vi "Open file.vi"(0 "reference in":refnum<class "TDMS_DataHandler.lvclass">, 5 "error in (no error)":errorcluster) -> (14 "reference out":refnum<class "TDMS_DataHandler.lvclass">, 15 "tdms file out":refnum<k34>, 19 "error out":errorcluster)   [LabVIEW 2019, in "TDMS_DataHandler.lvclass"]
uses:
  TDMS_DataHandler.lvclass
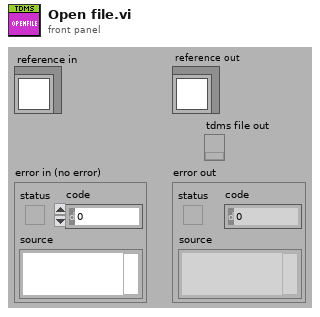
[diagram p1: front panel]
types:
  T1 = enum16{"open", "open or create", "create or replace", "create", "open (read-only)"}
  T2 = typedef "TDMS_DataHandler.lvclass/ObjectAttributesRef.ctl" = refnum<data-value>
  T3 = typedef "TDMS_DataHandler.lvclass/ObjectAttributes.ctl" = cluster{"Directory":path, "FilePath":path, "FileRef":refnum<k34>, "ExperimentName":string, "GroupName":string, "ChannelNames":string[], "Datum":waveform(dbl)[], "Group_Metadata":cluster{"property names":string[], "property values":variant[]}, "Channel_Metadata":cluster{"property names":string[], "property values":variant[]}}
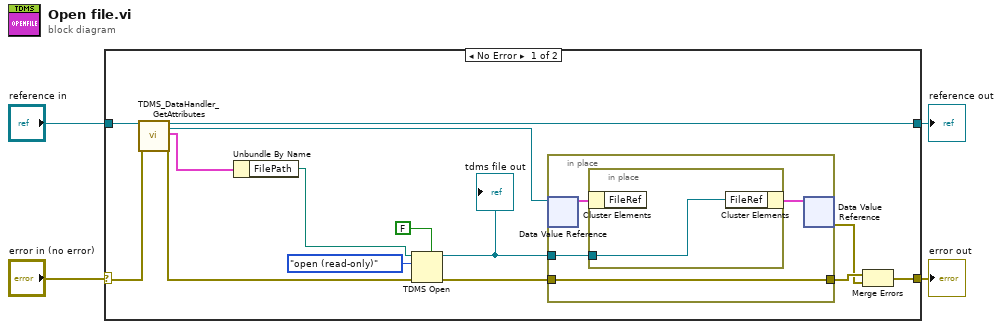
[diagram p0: block diagram]
diagram:
  n1 = case shown="No Error" "error in (no error)" {
    selector: "error in (no error)" -> [w16 w25]
    tunnel: [w18 w25] -> w3
    tunnel: [w11 w24] -> w1
    tunnel: "reference in" -> [w17 w24]
    frame No Error {
      n2 = call "TDMS_DataHandler_GetAttributes.vi"("reference in"=w17, "error in (no error)"=w16) -> ("reference out"=w11:refnum<class "TDMS_DataHandler.lvclass">, "attributes ref"=w13:T2, "attributes"=w12:T3, "error out"=w10:errorcluster)  [unwired: 14 in]
      n3 = Unbundle By Name(w12) -> ("FilePath"=w7:path)
      n4 = TDMS Open(5:FALSE ("create index file? (T)"), 8:w10, 10:T1."open (read-only)" ("operation (0:open)"), 11:w7) -> (0:w9:errorcluster, 3:w8:refnum<k34>)  [unwired: 3 in]
      "tdms file out" <- w8
      n5 = in-place {
        in-place-border: w9 -> [w20]
        in-place-border: [w20] -> w15
        in-place-border: w8 -> [w19]
        n6 = in-place-dvr #1(w13) -> (w21:T3)  [unwired: 1 out]
        n7 = in-place {
          in-place-border: w19 -> [w23]
          n8 = in-place-cluster #2(w21) -> ()  [unwired: 1 out]
          n9 = in-place-cluster #2("FileRef"=w23) -> (w22:T3)
        }
        n10 = in-place-dvr #1(w22) -> (w14:errorcluster)  [unwired: 1 out]
      }
      n11 = Merge Errors(w15, w14) -> (w18:errorcluster)
    }
    frame Error {
    }
  }
  "error out" <- w3
  "reference out" <- w1
